vi "emi_Splash&About Screen.vi"(0 "Parrent vi during starrt(Calling VI)":refnum<vi>, 3 "Fade/Rise time s(0)":dbl, 5 "error in (no error)":errorcluster, 6 "Action":T2(ring)=enum."Update", 7 "Status text":string, 9 "Optional App name":string="...") -> (19 "error out":errorcluster)   [LabVIEW 2011]
uses:
  Basic/0 - General/App/Version/Private/_emi_Version Holder.vi
  <vilib>/UserTags/UserTags.lvlib
panel:
  out "Initialization task":string
  out "Version Full":string="Version"
  out "App Name":string="Name"
  out "output cluster":T1
  out "Initializing":dbl(slide) step=2.84600433327e-312 scale=0.0..100.0
  # "Beagle"
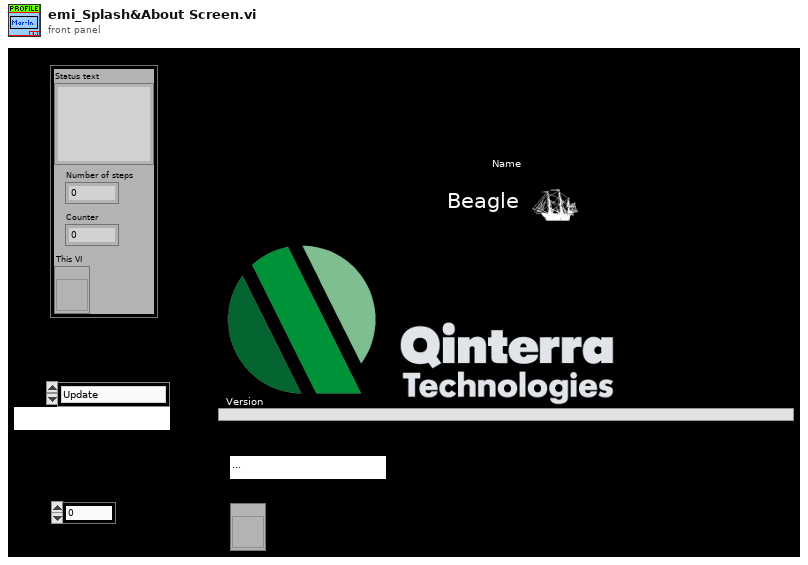
[diagram p1: front panel]
types:
  T1 = cluster{"Status text":string, "Number of steps":u16, "Counter":u16, "This VI":refnum<vi>}
  T2 = enum16{"Start", "Update", "End", "About Screen", "Just show"}
  T3 = enum32{"Invalid", "Default", "Floating", "Floating/Auto-Hide", "Modal"}
  T4 = typedef "emi_Version Info.ctl" = cluster{"Name":string, "Major":i16, "Minor":i16, "Fix":i16, "Build":i32, "Type":enum16{"Alfa", "Beta", "Stable"}, "Dev":bool, "Version Name":string, "Date":timestamp}
  T5 = enum32{"Invalid", "Standard", "Closed", "Hidden", "Minimized", "Maximized"}
  T6 = cluster{"Status text":string, "Numb Itt":i32, "Counter":u16, "This VI":refnum<vi>}
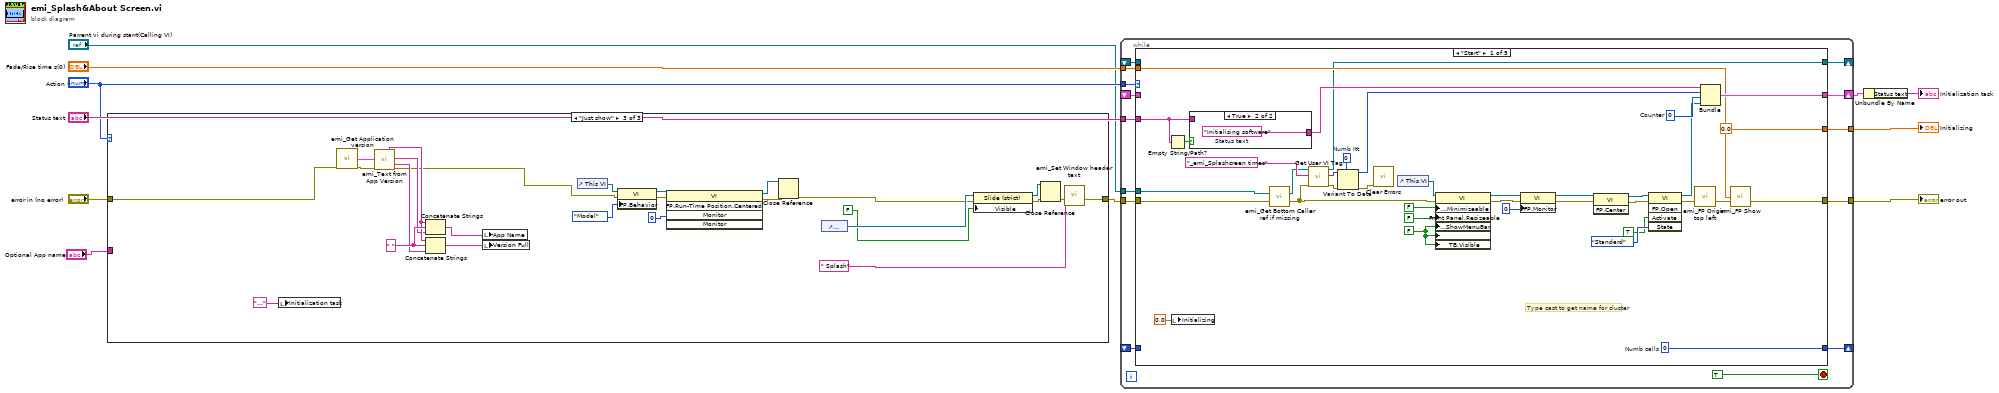
[diagram p0: block diagram]
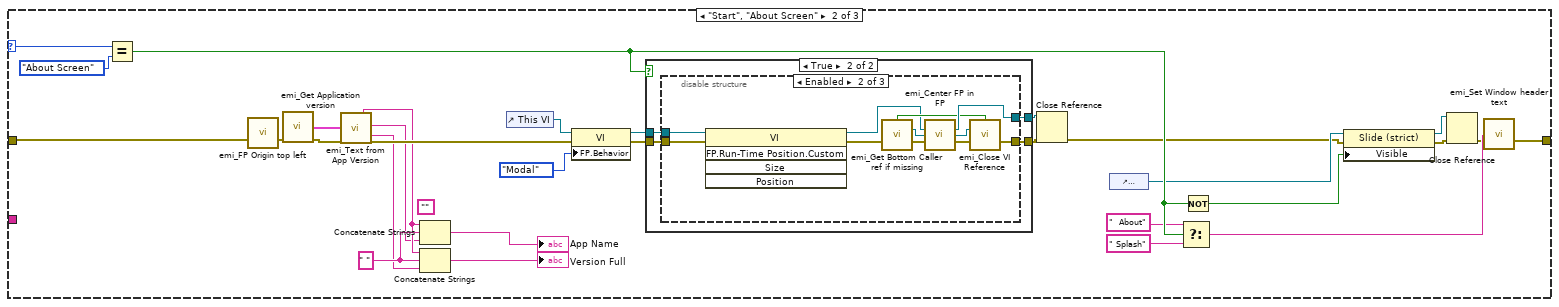
[diagram p3: hidden frame]
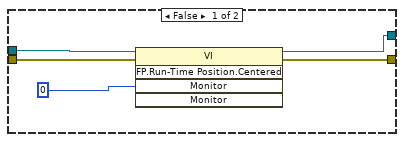
[diagram p4: hidden frame]
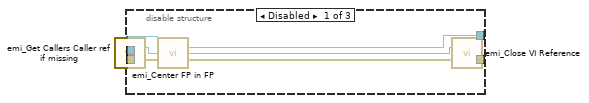
[diagram p5: hidden frame]
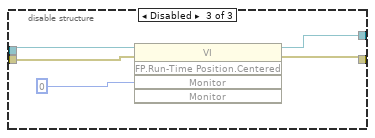
[diagram p6: hidden frame]
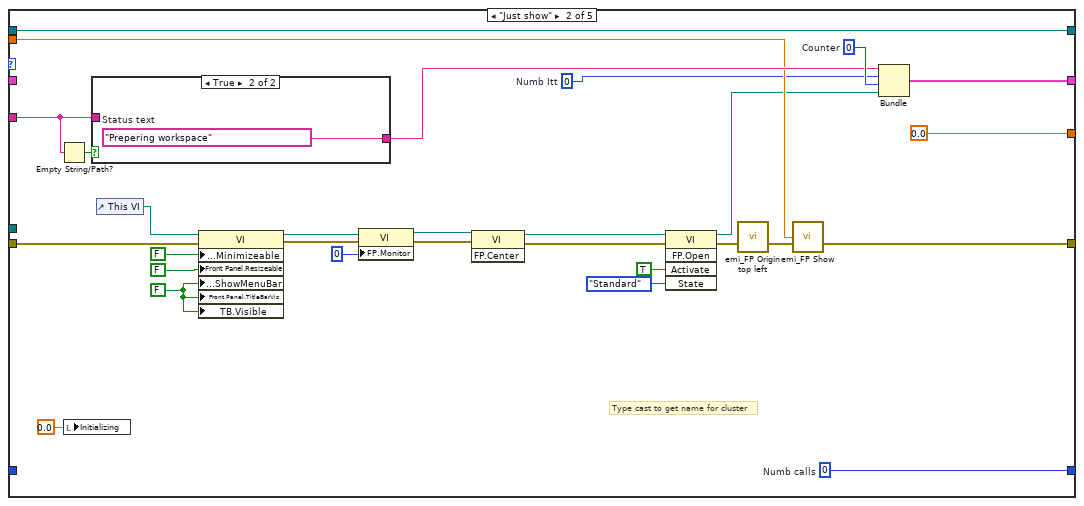
[diagram p8: hidden frame]
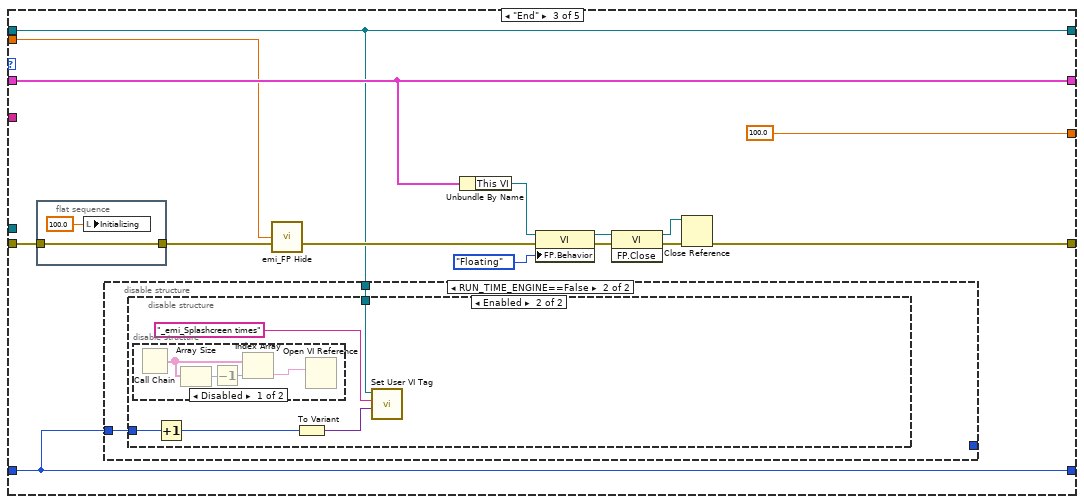
[diagram p10: hidden frame]
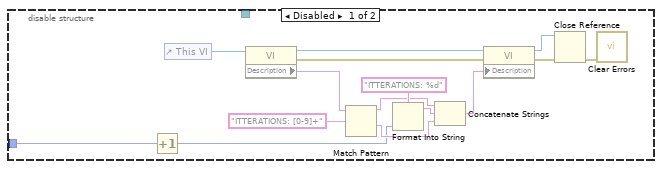
[diagram p12: hidden frame]
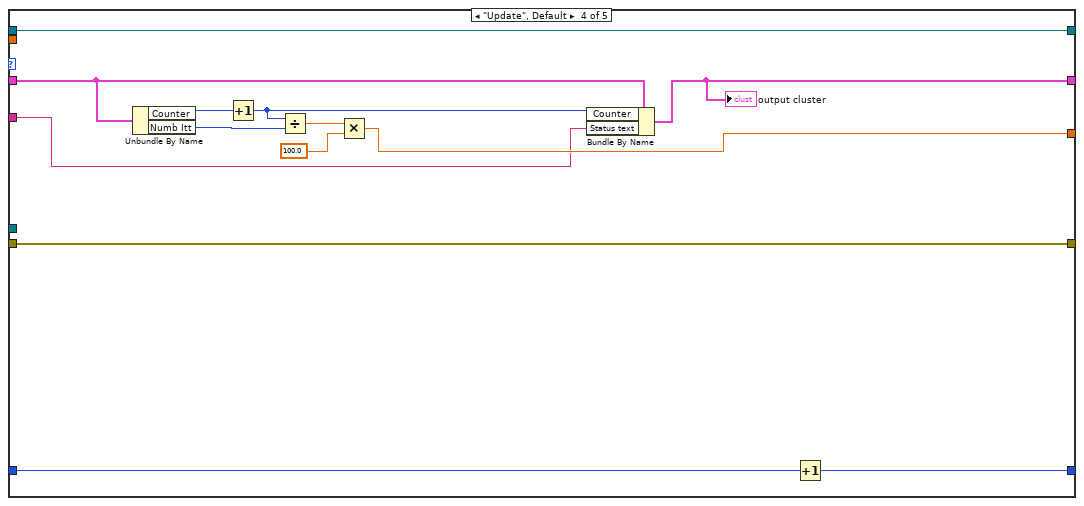
[diagram p14: hidden frame]
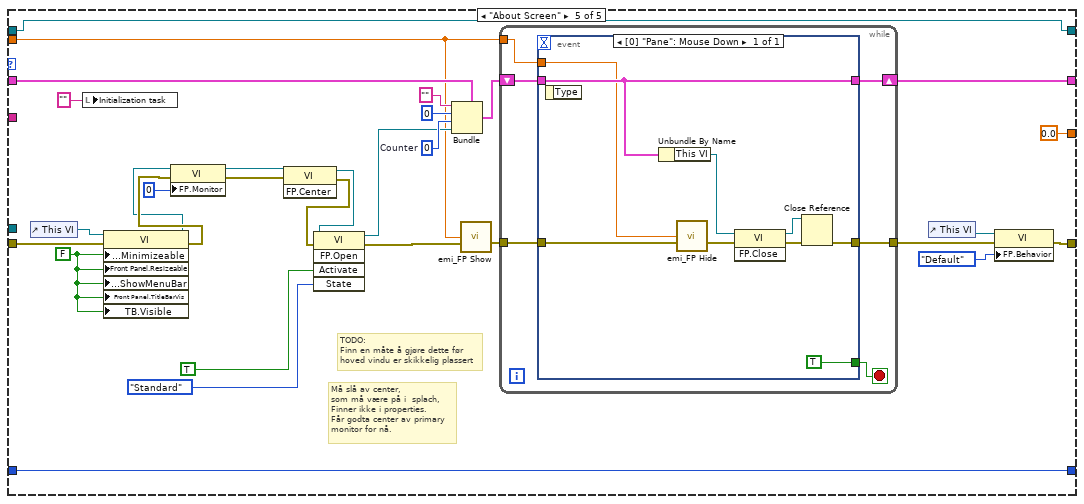
[diagram p15: hidden frame]
diagram:
  n1 = case shown="\"Just show\"" "Action" {
    selector: "Action" -> [_ w40 _]
    tunnel: "error in (no error)" -> [w12 w41 w80]
    tunnel: [w12 w42 w101] -> w5
    tunnel: "Optional App name" -> [_ _ _]
    frame Default {
    }
    frame "Start", "About Screen" {
      w17 = " " ("string")
      (unwired) ""
      n2 = Equal?(x=w40, y=T2."About Screen" ("Action")) -> (x = y?=w38:bool)
      n3 = call "emi_FP Origin top left.vi"("error in (no error)"=w41) -> ("error out"=w18:errorcluster)  [unwired: 13 in, 1 out]
      n4 = call "emi_Get Application version.vi"("error in (no error)"=w18) -> ("Version Info out"=w24:T4, "error out"=w25:errorcluster)  [unwired: 12 in, 1 out]
      n5 = call "emi_Text from App Version.vi"("Version Info"=w24, "error in (no error)"=w25) -> ("Name"=w16:string, "Short version Type"=w15:string, "Full version"=w14:string, "error out"=w19:errorcluster)  [unwired: 8 in, 6 out]
      n6 = Concatenate Strings(w16, w17, w15) -> (→"App Name":string)
      n7 = Concatenate Strings(w16, w17, w14) -> (→"Version Full":string)
      n8 = control-ref of="This VI"() -> (w27:refnum<vi>)
      n9 = property class="VI"(reference=w27, error in=w19, "FP.Behavior"=T3."Modal" ("Front Panel Window:Behavior")) -> (reference out=w22:refnum<vi>, error out=w23:errorcluster)
      n10 = case shown="True" w38 {
        tunnel: w23 -> [w47 w51]
        tunnel: w22 -> [w46 w50]
        tunnel: [w45 w49] -> w21
        tunnel: [w44 w48] -> w20
        frame False {
          n11 = invoke class="VI" method="FP.Run-Time Position.Centered"(reference=w46, error in=w47, "Monitor"=i16 0) -> (reference out=w45:refnum<vi>, error out=w44:errorcluster)  [unwired: 2 in, 3 out]
        }
        frame True {
          n12 = disable-structure shown="Enabled" {
            disable-tunnel: w51 -> [w58 w63 w74]
            disable-tunnel: w50 -> [w56 w62 w73]
            disable-tunnel: [w54 w70 w71] -> w49
            disable-tunnel: [w53 w67 w72] -> w48
            frame Disabled {
              n13 = call "emi_Get Callers Caller ref if missing.vi"("error in (no error)"=w58) -> ("VI Refnum Out"=w55:refnum<vi>, "error out"=w57:errorcluster)  [unwired: 12 in, 1 out]
              n14 = call "emi_Center FP in FP.vi"("VI To position Refnum(This vi)"=w56, "VI Anchor Refnum(Caller)"=w55, "error in (no error)"=w57) -> ("VI to Position Refnum"=w54:refnum<vi>, "VI Anchor Refnum"=w52:refnum<vi>, "error out"=w59:errorcluster)  [unwired: 10 in]
              n15 = call "emi_Close VI Reference.vi"("VI Refnum"=w52, "error in (no error)"=w59) -> ("error out"=w53:errorcluster)  [unwired: 12 in, 1 out]
            }
            frame Enabled {
              n16 = invoke class="VI" method="FP.Run-Time Position.Custom"(reference=w62, error in=w63) -> (reference out=w60:refnum<vi>, error out=w61:errorcluster)  [unwired: 3 in, 3 out]
              n17 = call "emi_Get Bottom Caller ref if missing.vi"("error in (no error)"=w61) -> ("Ref Generated"=w64:bool, "VI Refnum Out"=w66:refnum<vi>, "error out"=w69:errorcluster)  [unwired: 12 in]
              n18 = call "emi_Center FP in FP.vi"("VI To position Refnum(This vi)"=w60, "VI Anchor Refnum(Caller)"=w66, "error in (no error)"=w69) -> ("VI to Position Refnum"=w70:refnum<vi>, "VI Anchor Refnum"=w65:refnum<vi>, "error out"=w68:errorcluster)  [unwired: 10 in]
              n19 = call "emi_Close VI Reference.vi"("Close ref?(T)"=w64, "VI Refnum"=w65, "error in (no error)"=w68) -> ("error out"=w67:errorcluster)  [unwired: 11 in, 1 out]
            }
            frame Disabled {
              n20 = invoke class="VI" method="FP.Run-Time Position.Centered"(reference=w73, error in=w74, "Monitor"=i16 0) -> (reference out=w71:refnum<vi>, error out=w72:errorcluster)  [unwired: 2 in, 3 out]
            }
          }
        }
      }
      n21 = Close Reference(reference=w21, error in (no error)=w20) -> (error out=w13:errorcluster)
      n22 = control-ref of="Initializing"() -> (w31:refnum<vi>)
      n23 = Select(t="  About" ("string"), s=w38, f=" Splash" ("string")) -> (s? t:f=w32:string)
      n24 = Not(x=w38) -> (.not. x?=w35:bool)
      n25 = property class="Slide (strict)"(reference=w31, error in=w13, "Visible"=w35) -> (reference out=w28:refnum<vi>, error out=w30:errorcluster)
      n26 = Close Reference(reference=w28, error in (no error)=w30) -> (error out=w29:errorcluster)
      n27 = call "emi_Set Window header text.vi"("Header String"=w32, "error in (no error)"=w29) -> ("error out"=w42:errorcluster)  [unwired: 12 in, 1 out]
    }
    frame "Just show" {
      w84 = " " ("string")
      n28 = local write "Initialization task"("..." ("Initialization task")) -> ()
      n29 = call "emi_Get Application version.vi"("error in (no error)"=w80) -> ("Version Info out"=w85:T4, "error out"=w86:errorcluster)  [unwired: 12 in, 1 out]
      n30 = call "emi_Text from App Version.vi"("Version Info"=w85, "error in (no error)"=w86) -> ("Name"=w83:string, "Short version Type"=w82:string, "Full version"=w81:string, "error out"=w79:errorcluster)  [unwired: 8 in, 6 out]
      n31 = Concatenate Strings(w83, w84, w82) -> (w78:string)
      n32 = Concatenate Strings(w83, w84, w81) -> (w77:string)
      n33 = local write "App Name"(w78) -> ()
      n34 = local write "Version Full"(w77) -> ()
      n35 = control-ref of="This VI"() -> (w96:refnum<vi>)
      n36 = property class="VI"(reference=w96, error in=w79, "FP.Behavior"=T3."Modal" ("Front Panel Window:Behavior")) -> (reference out=w93:refnum<vi>, error out=w94:errorcluster)
      n37 = invoke class="VI" method="FP.Run-Time Position.Centered"(reference=w93, error in=w94, "Monitor"=i16 0) -> (reference out=w92:refnum<vi>, error out=w91:errorcluster)  [unwired: 2 in, 3 out]
      n38 = Close Reference(reference=w92, error in (no error)=w91) -> (error out=w76:errorcluster)
      n39 = control-ref of="Initializing"() -> (w100:refnum<vi>)
      n40 = property class="Slide (strict)"(reference=w100, error in=w76, "Visible"=FALSE) -> (reference out=w97:refnum<vi>, error out=w99:errorcluster)
      n41 = Close Reference(reference=w97, error in (no error)=w99) -> (error out=w98:errorcluster)
      n42 = call "emi_Set Window header text.vi"("Header String"=" Splash" ("string"), "error in (no error)"=w98) -> ("error out"=w101:errorcluster)  [unwired: 12 in, 1 out]
    }
  }
  n43 = while {
    tunnel: "Action" -> [w115]
    tunnel: w5 -> [w114]
    tunnel: [w113] -> w11
    shift-right: [w111] -> w10
    shift-left: _ -> [w110]
    tunnel: "Status text" -> [w109]
    tunnel: [w108] -> w7
    tunnel: "Fade/Rise time s(0)" -> [w107]
    shift-right: [w106] -> _
    shift-left: _ -> [w105]
    shift-right: [w104] -> _
    shift-left: _ -> [w103]
    tunnel: "Parrent vi during starrt(Calling VI)" -> [w102]
    stop <- TRUE stop-if-true
    n44 = case shown="\"Start\"" w115 {
      tunnel: [w149 w180 w198 w235 w258] -> w113
      tunnel: w114 -> [w129 w164 w196 w235 w271]
      tunnel: [w148 w179 w200 w239 w269] -> w111
      tunnel: w110 -> [_ _ w200 w240 w270]
      tunnel: w109 -> [w145 w176 _ w233 _]
      tunnel: [0.0 0.0 100.0 w234 0.0] -> w108
      tunnel: w107 -> [w141 w172 w195 _ w253]
      tunnel: [w140 w171 w187 w231 w263] -> w106
      tunnel: w105 -> [_ _ w187 w232 w263]
      tunnel: [w124 w162 w186 w230 w250] -> w104
      tunnel: w103 -> [_ w162 w186 w230 w250]
      tunnel: w102 -> [w123 _ _ _ _]
      frame "Start" {
        w131 = 0  # Numb Itt
        w140 = 0  # Numb calls
        w147 = u16 0  # Counter
        w152 = FALSE ("Front Panel Window:Resizeable")
        # "Type cast to get name for cluster"
        n45 = Empty String/Path?(string/path=w145) -> (empty?=w146:bool)
        n46 = local write "Initializing"(0.0 ("Initializing")) -> ()
        n47 = case shown="True" w146 {
          tunnel: w145 -> [w153 _]
          tunnel: [w153 w154] -> w144
          frame False {
          }
          frame True {
            w154 = "Initialising software"  # Status text
          }
        }
        n48 = call "emi_Get Bottom Caller ref if missing.vi"("VI Refnum(Calling VI)"=w123, "error in (no error)"=w129) -> ("VI Refnum Out"=w128:refnum<vi>, "error out"=w125:errorcluster)  [unwired: 11 in, 1 out]
        n49 = call <vilib>:"Get User VI Tag.vi"("error in (no error)"=w125, "Tag Name"="_emi_Splashcreen times", "VI Refnum"=w128) -> ("error out"=w134:errorcluster, "Value"=w132:variant, "dup VI Refnum"=w124:refnum<vi>)  [unwired: 5 in, 1 out]
        n50 = Variant To Data(error in=w134, type=w131, Variant=w132) -> (data=w130:i32, error out=w126:errorcluster)
        n51 = call <vilib>:"Clear Errors.vi"("error in (no error)"=w126) -> ()  [unwired: 6 in, 1 out]
        n52 = control-ref of="This VI"() -> (w135:refnum<vi>)
        n53 = property class="VI"(reference=w135, error in=w125, "Front Panel.Minimizeable"=FALSE ("Front Panel Window:Resizeable"), "Front Panel.Resizeable"=FALSE ("Front Panel Window:Resizeable"), "Front Panel.ShowMenuBar"=w152, "Front Panel.TitleBarVis"=w152, "TB.Visible"=w152) -> (reference out=w118:refnum<vi>, error out=w119:errorcluster)
        n54 = property class="VI"(reference=w118, error in=w119, "FP.Monitor"=u16 0 ("Front Panel Window:Monitor")) -> (reference out=w121:refnum<vi>, error out=w122:errorcluster)
        n55 = invoke class="VI" method="FP.Center"(reference=w121, error in=w122) -> (reference out=w116:refnum<vi>, error out=w117:errorcluster)  [unwired: 1 in, 1 out]
        n56 = invoke class="VI" method="FP.Open"(reference=w116, error in=w117, "Activate"=TRUE ("Activate?"), "State"=T5."Standard") -> (reference out=w127:refnum<vi>, error out=w136:errorcluster)  [unwired: 1 in, 3 out]
        n57 = call "emi_FP Origin top left.vi"("error in (no error)"=w136) -> ("error out"=w137:errorcluster)  [unwired: 13 in, 1 out]
        n58 = Bundle("Status text"=w144, "Numb Itt"=w130, "Counter"=w147, "This VI"=w127) -> (w148:T6)  [unwired: 1 in]
        n59 = call "emi_FP Show.vi"("Show time s(0)"=w141, "error in (no error)"=w137) -> ("error out"=w149:errorcluster)  [unwired: 12 in, 1 out]
      }
      frame "Just show" {
        w165 = 0  # Numb Itt
        w171 = 0  # Numb calls
        w178 = u16 0  # Counter
        w183 = FALSE ("Front Panel Window:Resizeable")
        # "Type cast to get name for cluster"
        n60 = Empty String/Path?(string/path=w176) -> (empty?=w177:bool)
        n61 = local write "Initializing"(0.0 ("Initializing")) -> ()
        n62 = case shown="True" w177 {
          tunnel: w176 -> [w184 _]
          tunnel: [w184 w185] -> w175
          frame False {
          }
          frame True {
            w185 = "Prepering workspace"  # Status text
          }
        }
        n63 = control-ref of="This VI"() -> (w166:refnum<vi>)
        n64 = property class="VI"(reference=w166, error in=w164, "Front Panel.Minimizeable"=FALSE ("Front Panel Window:Resizeable"), "Front Panel.Resizeable"=FALSE ("Front Panel Window:Resizeable"), "Front Panel.ShowMenuBar"=w183, "Front Panel.TitleBarVis"=w183, "TB.Visible"=w183) -> (reference out=w160:refnum<vi>, error out=w161:errorcluster)
        n65 = property class="VI"(reference=w160, error in=w161, "FP.Monitor"=u16 0 ("Front Panel Window:Monitor")) -> (reference out=w158:refnum<vi>, error out=w159:errorcluster)
        n66 = invoke class="VI" method="FP.Center"(reference=w158, error in=w159) -> (reference out=w156:refnum<vi>, error out=w157:errorcluster)  [unwired: 1 in, 1 out]
        n67 = invoke class="VI" method="FP.Open"(reference=w156, error in=w157, "Activate"=TRUE ("Activate?"), "State"=T5."Standard") -> (reference out=w163:refnum<vi>, error out=w167:errorcluster)  [unwired: 1 in, 3 out]
        n68 = call "emi_FP Origin top left.vi"("error in (no error)"=w167) -> ("error out"=w168:errorcluster)  [unwired: 13 in, 1 out]
        n69 = call "emi_FP Show.vi"("Show time s(0)"=w172, "error in (no error)"=w168) -> ("error out"=w180:errorcluster)  [unwired: 12 in, 1 out]
        n70 = Bundle("Status text"=w175, "Numb Itt"=w165, "Counter"=w178, "This VI"=w163) -> (w179:T6)  [unwired: 1 in]
      }
      frame "End" {
        n71 = flat-sequence {
          tunnel: [w228] -> w197
          tunnel: w196 -> [w228]
          frame #0 {
            n72 = local write "Initializing"(100.0 ("Initializing")) -> ()
          }
        }
        n73 = disable-structure shown="RUN_TIME_ENGINE==False" {
          disable-tunnel: w187 -> [w201 w203]
          disable-tunnel: [w201 _] -> _
          disable-tunnel: w186 -> [_ w202]
          frame condition #0 {
          }
          frame condition #1 (active) {
            n74 = disable-structure shown="Enabled" {
              disable-tunnel: w203 -> [w211 w221]
              disable-tunnel: w202 -> [_ w219]
              frame Disabled {
                n75 = Increment(x=w211) -> (x+1=w204:i32)
                n76 = control-ref of="This VI"() -> (w218:refnum<vi>)
                n77 = property class="VI"(reference=w218) -> (reference out=w217:refnum<vi>, error out=w205:errorcluster, "Description"=w213:string)  [unwired: 1 in]
                n78 = Match Pattern(string=w213, regular expression="ITTERATIONS: [0-9]+") -> (before substring=w209:string, after substring=w207:string)  [unwired: 1 in, 2 out]
                n79 = Format Into String(format string="ITTERATIONS: %d", w204) -> (resulting string=w208:string)  [unwired: 2 in, 1 out]
                n80 = Concatenate Strings(w209, w208, w207) -> (w206:string)
                n81 = property class="VI"(reference=w217, error in=w205, "Description"=w206) -> (reference out=w214:refnum<vi>, error out=w216:errorcluster)
                n82 = Close Reference(reference=w214, error in (no error)=w216) -> (error out=w215:errorcluster)
                n83 = call <vilib>:"Clear Errors.vi"("error in (no error)"=w215) -> ()  [unwired: 6 in, 1 out]
              }
              frame Enabled {
                n84 = disable-structure shown="Disabled" {
                  frame Disabled {
                    n85 = Call Chain() -> (call chain=w226:string[])
                    n86 = Array Size(array=w226) -> (size(s)=w227:i32)
                    n87 = Decrement(x=w227) -> (x-1=w225:i32)
                    n88 = Index Array(array=w226, index=w225) -> (element=w224:string)
                    n89 = Open VI Reference(vi path=w224) -> ()  [unwired: 1 in, 6 out]
                  }
                  frame Enabled {
                  }
                }
                n90 = Increment(x=w221) -> (x+1=w220:i32)
                n91 = To Variant(anything=w220) -> (Variant=w222:variant)
                n92 = call <vilib>:"Set User VI Tag.vi"("Value"=w222, "Tag Name"="_emi_Splashcreen times", "VI Refnum"=w219) -> ()  [unwired: 6 in, 3 out]
              }
            }
          }
        }
        n93 = call "emi_FP Hide.vi"("Show time s(0)"=w195, "error in (no error)"=w197) -> ("error out"=w189:errorcluster)  [unwired: 12 in, 1 out]
        n94 = Unbundle By Name(w200) -> ("This VI"=w190:refnum<vi>)
        n95 = property class="VI"(reference=w190, error in=w189, "FP.Behavior"=T3."Floating" ("Front Panel Window:Behavior")) -> (reference out=w192:refnum<vi>, error out=w191:errorcluster)
        n96 = invoke class="VI" method="FP.Close"(reference=w192, error in=w191) -> (reference out=w194:refnum<vi>, error out=w193:errorcluster)  [unwired: 1 in, 1 out]
        n97 = Close Reference(reference=w194, error in (no error)=w193) -> (error out=w198:errorcluster)
      }
      frame "Update", Default {
        n98 = Unbundle By Name(w240) -> ("Counter"=w238:u16, "Numb Itt"=w236:i32)
        n99 = Increment(x=w238) -> (x+1=w237:u16)
        n100 = Divide(x=w237, y=w236) -> (x/y=w242:dbl)
        n101 = Multiply(x=w242, y=100.0 ("x")) -> (x*y=w234:dbl)
        n102 = Bundle By Name(cluster=w240, "Counter"=w237, "Status text"=w233) -> (w239:T6)
        "output cluster" <- w239
        n103 = Increment(x=w232) -> (x+1=w231:i32)
      }
      frame "About Screen" {
        w266 = u16 0  # Counter
        w257 = FALSE ("Front Panel Window:Resizeable")
        # "Må slå av center, \nsom må være på i  splach,\nFinner ikke i properties.\nFår godta center av primary \nmonitor for nå."
        # "TODO:\nFinn en måte å gjøre dette før \nhoved vindu er skikkelig plassert"
        n104 = control-ref of="This VI"() -> (w268:refnum<vi>)
        n105 = local write "Initialization task"("" ("Initialization task")) -> ()
        n106 = property class="VI"(reference=w268, error in=w271, "Front Panel.Minimizeable"=w257, "Front Panel.Resizeable"=w257, "Front Panel.ShowMenuBar"=w257, "Front Panel.TitleBarVis"=w257, "TB.Visible"=w257) -> (reference out=w245:refnum<vi>, error out=w246:errorcluster)
        n107 = property class="VI"(reference=w245, error in=w246, "FP.Monitor"=u16 0 ("Front Panel Window:Monitor")) -> (reference out=w248:refnum<vi>, error out=w249:errorcluster)
        n108 = invoke class="VI" method="FP.Center"(reference=w248, error in=w249) -> (reference out=w243:refnum<vi>, error out=w244:errorcluster)  [unwired: 1 in, 1 out]
        n109 = invoke class="VI" method="FP.Open"(reference=w243, error in=w244, "Activate"=TRUE ("Activate?"), "State"=T5."Standard") -> (reference out=w254:refnum<vi>, error out=w252:errorcluster)  [unwired: 1 in, 3 out]
        n110 = Bundle(cluster=w270, "Status text"="", "Numb Itt"=0, "Counter"=w266, "This VI"=w254) -> (w265:T6)
        n111 = call "emi_FP Show.vi"("Show time s(0)"=w253, "error in (no error)"=w252) -> ("error out"=w251:errorcluster)  [unwired: 12 in, 1 out]
        n112 = while {
          tunnel: [w278] -> w259
          tunnel: w251 -> [w276]
          shift-right: [w277] -> w269
          shift-left: w265 -> [w275]
          tunnel: w253 -> [w273]
          stop <- w274 stop-if-true
          n113 = event shown="[0] \"Pane\": Mouse Down" {
            selector: _ -> [_]
            dyn-events: _ -> [_]
            timeout: _ -> [_]
            tunnel: [w282] -> w278
            tunnel: w276 -> [w279]
            tunnel: w275 -> [w281]
            tunnel: [w281] -> w277
            tunnel: [TRUE] -> w274
            tunnel: w273 -> [w280]
            event Mouse Down {
              n114 = event-data() -> ()  [unwired: 1 in, 1 out]
              n115 = Unbundle By Name(w281) -> ("This VI"=w286:refnum<vi>)
              n116 = call "emi_FP Hide.vi"("Show time s(0)"=w280, "error in (no error)"=w279) -> ("error out"=w283:errorcluster)  [unwired: 12 in, 1 out]
              n117 = invoke class="VI" method="FP.Close"(reference=w286, error in=w283) -> (reference out=w285:refnum<vi>, error out=w284:errorcluster)  [unwired: 1 in, 1 out]
              n118 = Close Reference(reference=w285, error in (no error)=w284) -> (error out=w282:errorcluster)
            }
          }
        }
        n119 = control-ref of="This VI"() -> (w261:refnum<vi>)
        n120 = property class="VI"(reference=w261, error in=w259, "FP.Behavior"=T3."Default" ("Front Panel Window:Behavior")) -> (error out=w258:errorcluster)  [unwired: 1 out]
      }
    }
  }
  "error out" <- w11
  "Initializing" <- w7
  n121 = Unbundle By Name(w10) -> ("Status text"=→"Initialization task":string)
